vi "S7 TCP Test2.vi"() -> ()   [LabVIEW 2014]
uses:
  S7 TCP API Library/S7 Read Write Cluster.ctl
  S7 TCP API Library/Data Type.ctl
  S7 TCP API Library/S7 TCP.lvlib
panel:
  in  "IP Address":string="172.16.102.180"
  out "Loop Time":dbl
  in  "milliseconds to wait":u32=100
  out "Data Valid Array":bool[](array[boolean])
  out "Output Data":dbl[](array[numeric])
  in  "S7 Read Write Array":T1[](array[typedef])=[{"Read / Write"=4, "Address Areas"=132, "Data Block #"=0, "Start Address (bytes)"=10, "Data Type"=enum."Word (U16)", "Bit Number / Byte Length"=0, "Write Data"=0.0}, {"Read / Write"=4, "Address Areas"=132, "Data Block #"=0, "Start Address (bytes)"=201, "Data Type"=enum."Bit", "Bit Number / Byte Length"=7, "Write Data"=0.0}, {"Read / Write"=4, "Address Areas"=132, "Data Block #"=0, "Start Address (bytes)"=201, "Data Type"=enum."Byte (U8)", "Bit Number / Byte Length"=0, "Write Data"=0.0}, {"Read / Write"=4, "Address Areas"=132, "Data Block #"=0, "Start Address (bytes)"=201, "Data Type"=enum."Real (SGL)", "Bit Number / Byte Length"=0, "Write Data"=0.0}, {"Read / Write"=4, "Address Areas"=132, "Data Block #"=1, "Start Address (bytes)"=201, "Data Type"=enum."Byte (U8)", "Bit Number / Byte Length"=0, "Write Data"=0.0}, {"Read / Write"=4, "Address Areas"=132, "Data Block #"=1, "Start Address (bytes)"=201, "Data Type"=enum."Signed Byte (I8)", "Bit Number / Byte Length"=0, "Write Data"=0.0}] {"Address Areas" items=["I/O (P)"=128, "Input (I)"=129, "Output (Q)"=130, "Bit Memory (M)"=131, "Data (DB)"=132, "Instance Data (DI)"=133, "Local Data (L)"=134, "Predecessor Local Data (VL)"=135]; "Read / Write" items=["Read"=4, "Write"=5]; "Bit Number / Byte Length" max=7 step=1}
  out "Loop Itteration":i32
  in  "Stop":bool
  out "error out":errorcluster
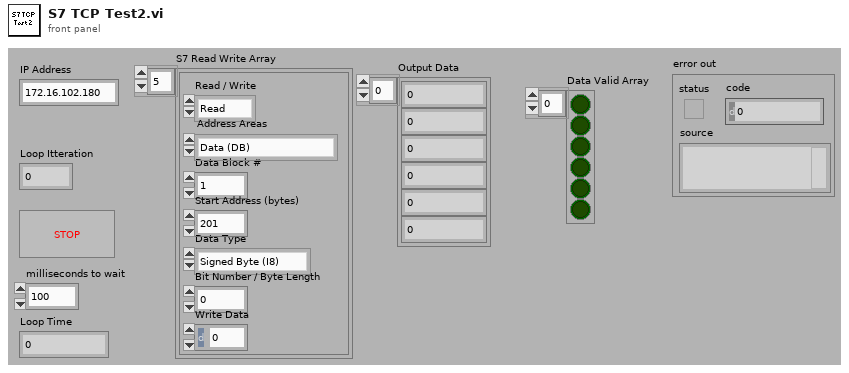
[diagram p1: front panel]
types:
  T1 = typedef "S7 TCP.lvlib/S7 Read Write Cluster.ctl" = cluster{"Read / Write":u8, "Address Areas":u8, "Data Block #":u16, "Start Address (bytes)":u32, "Data Type":T2, "Bit Number / Byte Length":u8, "Write Data":dbl}
  T2 = typedef "S7 TCP.lvlib/Data Type.ctl" = enum16{"Bit", "Byte (U8)", "Signed Byte (I8)", "Word (U16)", "Signed Word (I16)", "Long (U32)", "Signed Long (I32)", "Real (SGL)", "Defined Byte Length"}
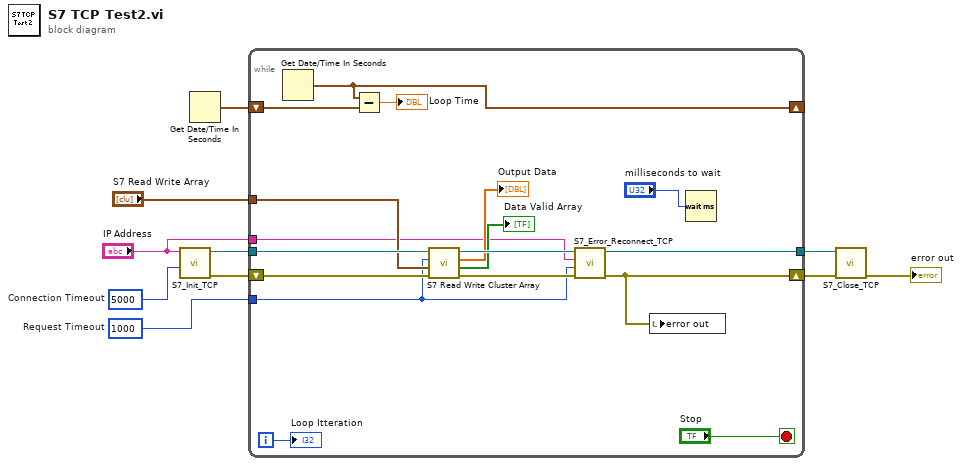
[diagram p0: block diagram]
diagram:
  w4 = u32 1000  # Request Timeout
  w8 = u32 5000  # Connection Timeout
  n1 = call "S7_Init_TCP.vi"("Connection Timeout"=w8, "IP Address"="IP Address") -> ("error out"=w6:errorcluster, "TCP Connection Ref"=w5:refnum<k5>)  [unwired: 3 in, 5 out]
  n2 = Get Date/Time In Seconds() -> (seconds since 1Jan1904=w3:timestamp)
  n3 = while {
    tunnel: w5 -> [w22]
    tunnel: [w24] -> w10
    tunnel: w4 -> [w12]
    shift-right: [w25] -> w7
    shift-left: w6 -> [w20]
    shift-right: [w15] -> _
    shift-left: w3 -> [w16]
    tunnel: "S7 Read Write Array" -> [w13]
    tunnel: "IP Address" -> [w11]
    i -> [w26]
    stop <- "Stop" stop-if-true
    n4 = Get Date/Time In Seconds() -> (seconds since 1Jan1904=w15:timestamp)
    n5 = Subtract(x=w15, y=w16) -> (x-y=→"Loop Time":dbl)
    n6 = call "S7 Read Write Cluster Array.vi"("error in"=w20, "S7 Read Write Array"=w13, "Timeout"=w12, "TCP Connection Ref"=w22) -> ("error out"=w19:errorcluster, "Data Valid Array"=→"Data Valid Array":bool[], "Output Data"=→"Output Data":dbl[], "TCP Connection Ref Out"=w21:refnum<k5>)  [unwired: 4 out]
    n7 = call "S7_Error_Reconnect_TCP.vi"("error in"=w19, "Timeout"=w12, "IP Address"=w11, "TCP Connection Ref"=w21) -> ("error out"=w25:errorcluster, "TCP Connection Ref Out"=w24:refnum<k5>)  [unwired: 6 out]
    n8 = local write "error out"(w25) -> ()
    n9 = Wait (ms)(milliseconds to wait="milliseconds to wait") -> ()  [unwired: 1 out]
    "Loop Itteration" <- w26
  }
  n10 = call "S7_Close_TCP.vi"("error in"=w7, "TCP Connection Ref"=w10) -> ("error out"=→"error out":errorcluster)  [unwired: 1 in, 8 out]
